vi "GaussianPeakFinder.vi"(3 "Mode":T4, 5 "Traverse line In":T1 {"Row Duration (mins)" format="%#.1f"; "Row No" min=0; "Trace Gas Concentration (%)" min=0.0 format="%#.2f"; "Emission Rate (l/min)" format="%#.2f"; "Tunnel Speed" format="%#.2f"; "Start X" format="%#.2f"; "Start Y" format="%#.2f"; "Start Z" format="%#.2f"; "End X" format="%#.2f"; "End Y" format="%#.2f"; "End Z" format="%#.2f"; "Averaging time (min)" min=0.0 format="%#.2f"}) -> (0 "Error Message":string, 1 "Status":T5, 2 "Traverse line Out":T1 {"Row Duration (mins)" format="%#.1f"; "Row No" min=0; "Trace Gas Concentration (%)" min=0.0 format="%#.2f"; "Emission Rate (l/min)" format="%#.2f"; "Tunnel Speed" format="%#.2f"; "Start X" format="%#.2f"; "Start Y" format="%#.2f"; "Start Z" format="%#.2f"; "End X" format="%#.2f"; "End Y" format="%#.2f"; "End Z" format="%#.2f"; "Averaging time (min)" min=0.0 format="%#.2f"})   [LabVIEW 2011]
uses:
  Gen Trav/Traverse_cluster.ctl
  Gen Trav/Spacing.ctl
  Controls/Multi_run_mode.ctl
  Controls/User_Specific_mode.ctl
  Gen Trav/Multi_Run_Status.ctl
  Controls/Save_Data.ctl
  Controls/Setup.ctl
  Utilities/gaussianFit/GaussianGlobal.vi
panel:
  in  "Tab Control":enum32{"GaussianFitGraph", "RunVINamed"}(tab)
  in  "nPointsInRake":i32=3
  out "nPointsSampled":i32
  in  "SpreadFactor":dbl=0.8
  in  "Turbulence":dbl=0.2
  in  "SampleLengthMultiplier":dbl=2.5
  out "MeasurementCenter":dbl
  # "X           Y            Z"
  # "Start"
  # "End"
  # "X           Y            Z"
  # "Start"
  # "End"
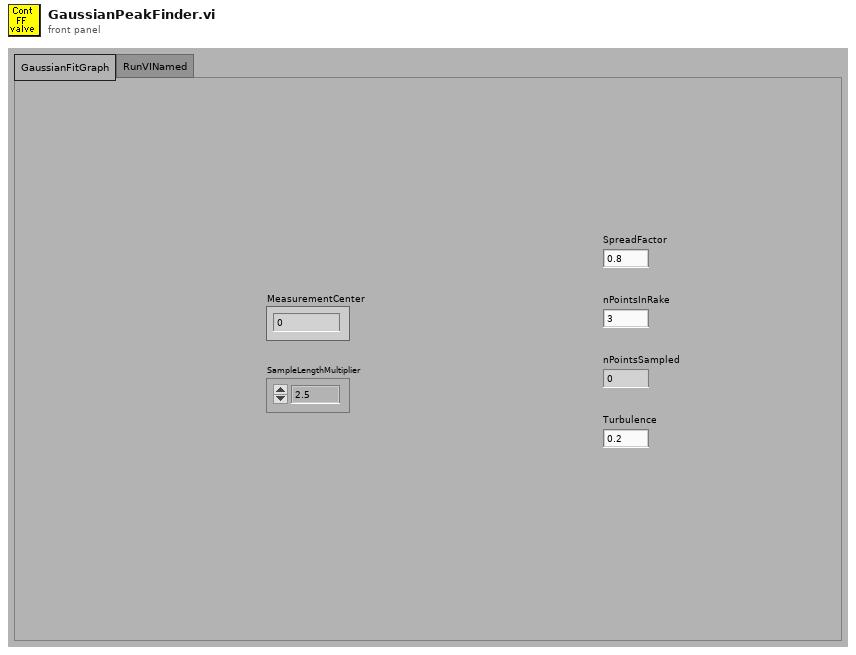
[diagram p1: front panel]
types:
  T1 = typedef "Traverse_cluster.ctl" = cluster{"Start X":dbl, "Start Y":dbl, "Start Z":dbl, "End X":dbl, "End Y":dbl, "End Z":dbl, "No. of pts.":i32, "Spacing":T2, "Filename":path, "Tunnel Speed":dbl, "Averaging time (min)":dbl, "Extra Commands":string, "Specific Arguments":string, "Emission Rate (l/min)":dbl, "Trace Gas Concentration (%)":dbl, "Density Ratio":string, "Comments":string, "Row No":i32, "Row Type Selector":T3, "Completion time":string, "Row Duration (mins)":dbl, "No. of Valid pts.":i32, "Meas Setup File":string}
  T2 = typedef "Spacing.ctl" = enum16{"Linear", "Log", "Gauss", "Specified", "N/A"}
  T3 = typedef "Multi_run_mode.ctl" = enum16{"Move Traverse Only", "Set Tunnel Speed Only", "Set Source Only", "Set Measurement Conditions", "Single Measurement", "Vertical Profile", "Lateral Profile", "Longitudinal Profile", "Explore Volume", "Multi-Axis Profile", "Auto Calibrate", "Meas Fast FID Bkgnd", "Check Beam Power", "Scanning Valve Measurement", "Run VI Named:", "Set ADAM Ch", "Wait (minutes)", "Send Message", "Synchronize With:", "Fall Back to this Row", "Turn Off Row Repeating", "Blank Row", "Traverse 3D Volume"}
  T4 = typedef "User_Specific_mode.ctl" = enum16{"Check VI only", "Run VI"}
  T5 = typedef "Multi_Run_Status.ctl" = enum16{"Continue", "Jump to Next Point", "Jump to Next Row", "Jump To Fall Back", "Terminate Run"}
  T6 = typedef "Save_Data.ctl" = enum16{"Save No Data", "Save Data"}
  T7 = typedef "Setup.ctl" = enum16{"Run Program", "Show Setup", "Save Current Setup", "Setup Front Panel"}
  T8 = typedef "Status_Cluster.ctl" = cluster{"Status":T5, "Error Type":string, "Error Description":string}
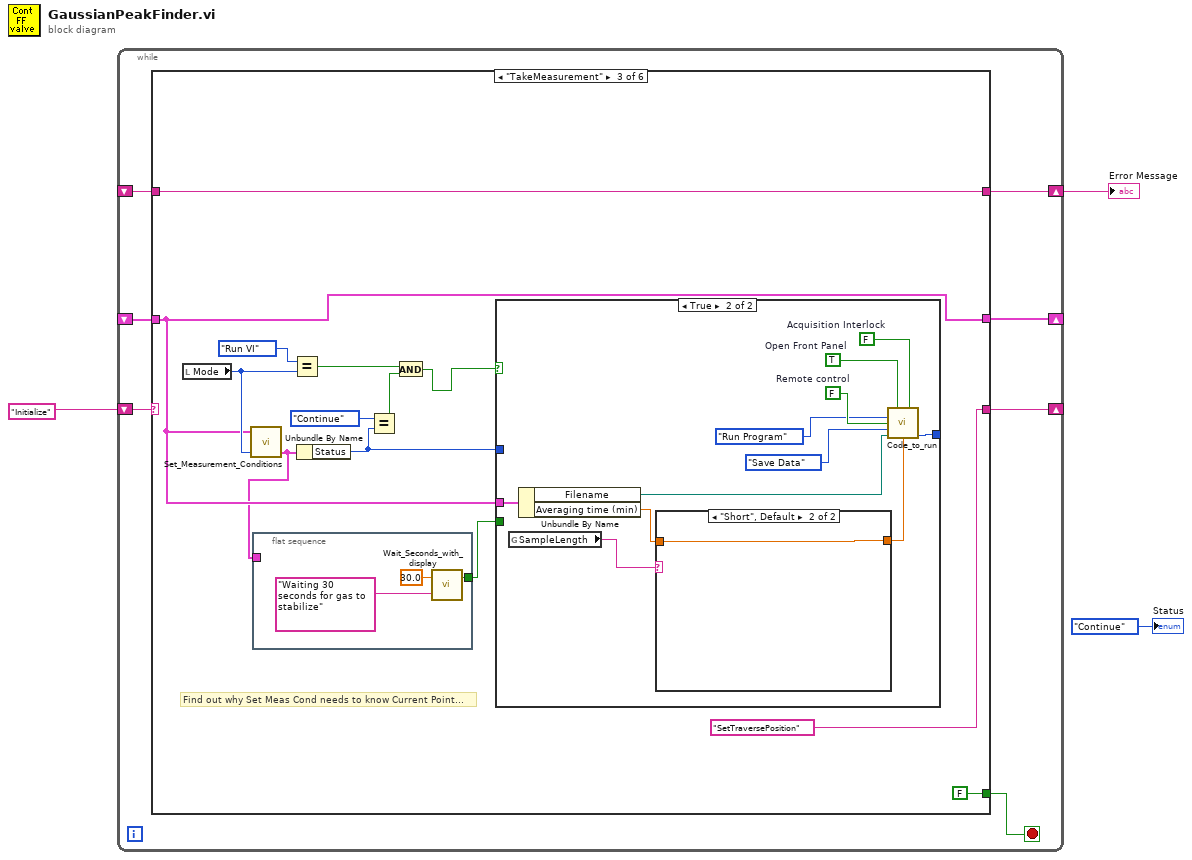
[diagram p0: block diagram]
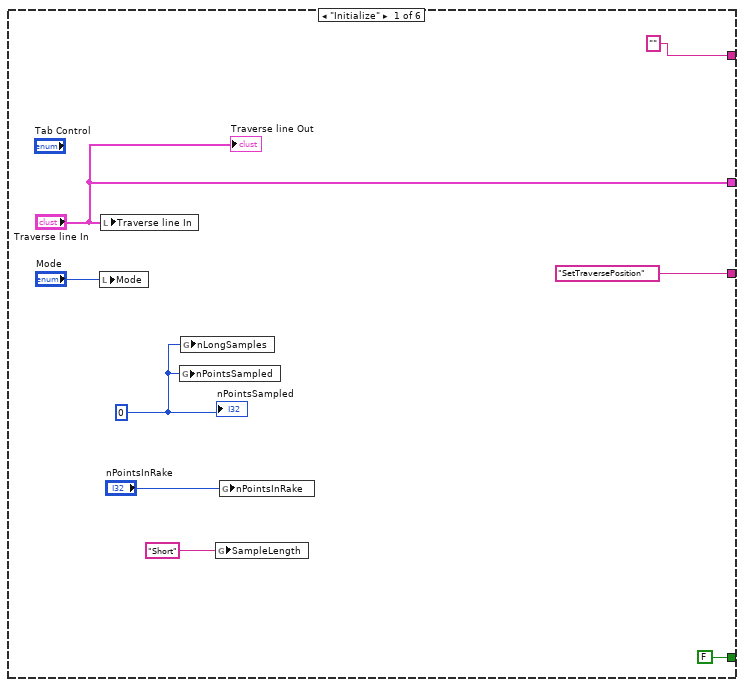
[diagram p2: hidden frame]
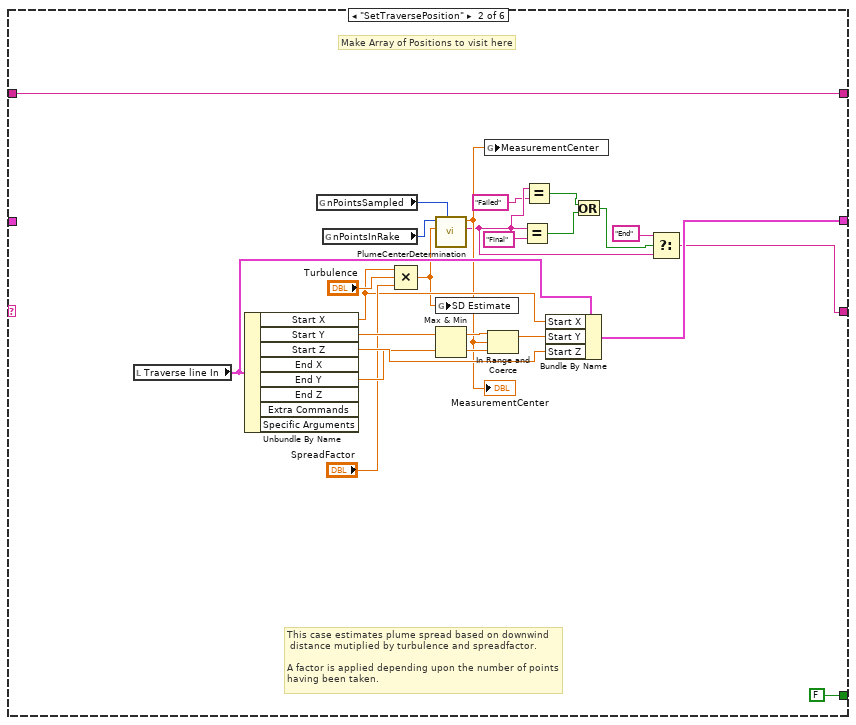
[diagram p3: hidden frame]
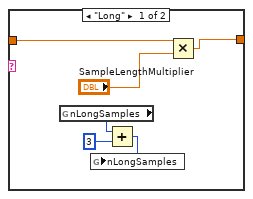
[diagram p5: hidden frame]
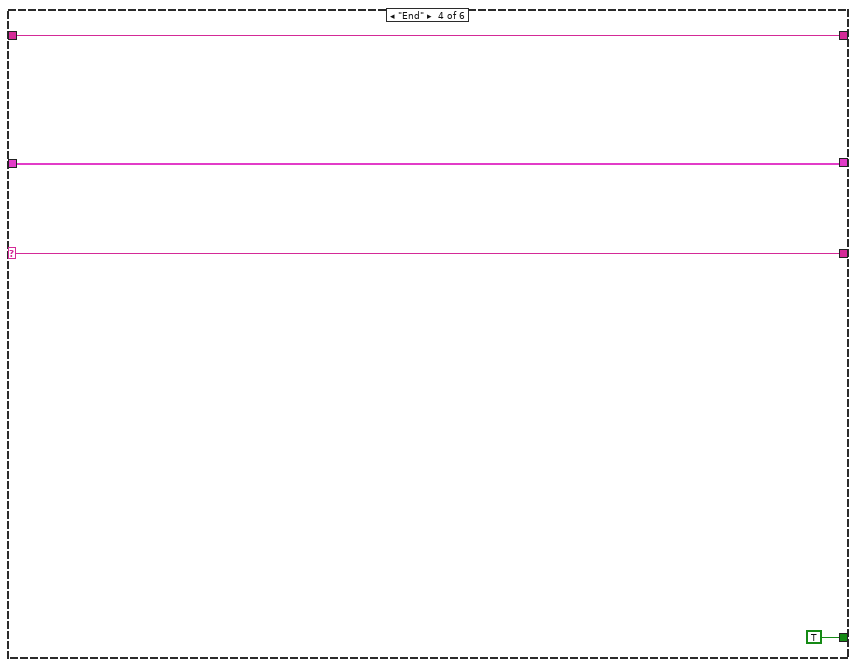
[diagram p6: hidden frame]
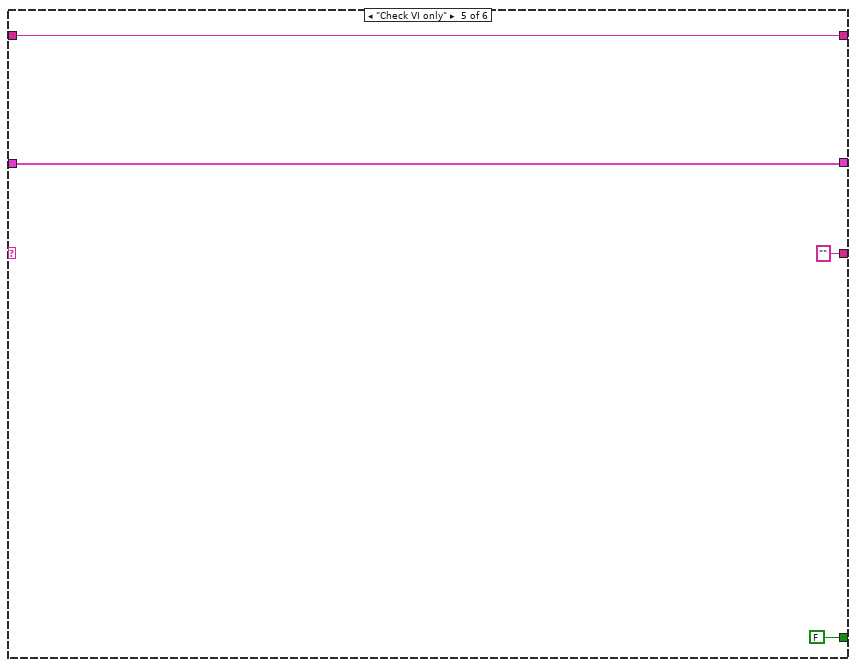
[diagram p7: hidden frame]
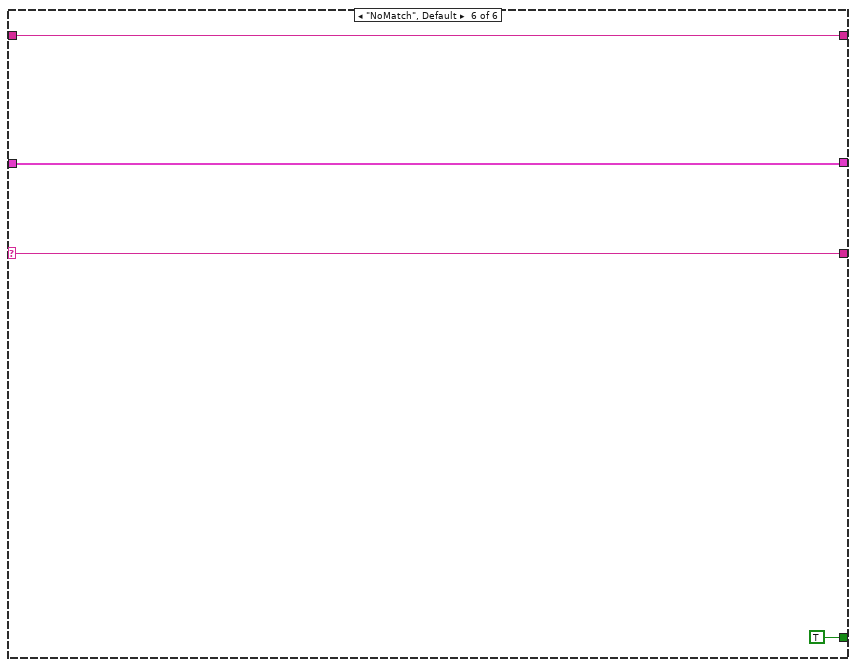
[diagram p8: hidden frame]
diagram:
  n1 = while {
    shift-right: [w8] -> _
    shift-left: _ -> [w7]
    shift-right: [w10] -> w2
    shift-left: _ -> [w5]
    shift-right: [w4] -> _
    shift-left: "Initialize" -> [w9]
    stop <- w6 stop-if-true
    n2 = case shown="\"TakeMeasurement\"" w9 {
      selector: w9 -> [_ _ _ w79 _ w87]
      tunnel: ["" w39 w50 w81 w84 w88] -> w10
      tunnel: ["Traverse line In" w42 w49 w80 w85 w89] -> w8
      tunnel: w7 -> [_ _ w49 w80 w85 w89]
      tunnel: [FALSE FALSE FALSE TRUE FALSE TRUE] -> w6
      tunnel: w5 -> [_ w39 w50 w81 w84 w88]
      tunnel: ["SetTraversePosition" w26 "SetTraversePosition" w79 "" w87] -> w4
      frame "Initialize" {
        w11 = 0 ("PointsSampled")
        n3 = local write "Mode"("Mode") -> ()
        n4 = local write "Traverse line In"("Traverse line In") -> ()
        n5 = global write "GaussianGlobal.vi" "nPointsSampled"(w11) -> ()
        n6 = global write "GaussianGlobal.vi" "nLongSamples"(w11) -> ()
        n7 = global write "GaussianGlobal.vi" "SampleLength"("Short" ("SampleLength")) -> ()
        n8 = global write "GaussianGlobal.vi" "nPointsInRake"("nPointsInRake") -> ()
        "nPointsSampled" <- w11
        "Traverse line Out" <- "Traverse line In"
      }
      frame "SetTraversePosition" {
        # "This case estimates plume spread based on downwind\n distance mutiplied by turbulence and spreadfactor.\n\nA factor is applied depending upon the number of points\nhaving been taken."
        # "Make Array of Positions to visit here"
        n9 = local read "Traverse line In"() -> (w41:T1)
        n10 = Unbundle By Name(w41) -> ("Start X"=w31:dbl, "Start Y"=w38:dbl, "Start Z"=w43:dbl, "End Y"=w37:dbl)  [unwired: 4 out]
        n11 = global read "GaussianGlobal.vi" "nPointsSampled"() -> (w29:i32)
        n12 = global read "GaussianGlobal.vi" "nPointsInRake"() -> (w30:i32)
        n13 = Compound Arithmetic op=MULTIPLY(w31, "Turbulence", "SpreadFactor") -> (w24:dbl)
        n14 = call "PlumeCenterDetermination.vi"("nPointsSampled"=w29, "SD Estimate"=w24, "nPointsInRake"=w30) -> ("CommandString"=w23:string, "Measurement Center"=w25:dbl)  [unwired: 7 in]
        "MeasurementCenter" <- w25
        n15 = global write "GaussianGlobal.vi" "SD Estimate"(w24) -> ()
        n16 = Max & Min(x=w38, y=w37) -> (max(x,y)=w36:dbl, min(x,y)=w35:dbl)
        n17 = global write "GaussianGlobal.vi" "MeasurementCenter"(w25) -> ()
        n18 = In Range and Coerce(upper limit=w36, x=w25, lower limit=w35) -> (coerced(x)=w34:dbl)  [unwired: 1 out]
        n19 = Equal?(x=w23, y="Final") -> (x = y?=w20:bool)
        n20 = Equal?(x=w23, y="Failed") -> (x = y?=w21:bool)
        n21 = Bundle By Name(cluster=w41, "Start X"=w31, "Start Y"=w34, "Start Z"=w43) -> (w42:T1)
        n22 = Or(x=w21, y=w20) -> (x .or. y?=w19:bool)
        n23 = Select(t="End" ("y"), s=w19, f=w23) -> (s? t:f=w26:string)
      }
      frame "TakeMeasurement" {
        # "Find out why Set Meas Cond needs to know Current Point..."
        n24 = local read "Mode"() -> (w52:T4)
        n25 = call "Set_Measurement_Conditions.vi"("Simulate/Run"=w52, "Traverse line"=w49) -> ("Status Cluster"=w44:T8)  [unwired: 3 in]
        n26 = flat-sequence {
          tunnel: [w59] -> w46
          tunnel: w44 -> [_]
          frame #0 {
            n27 = call "Wait_Seconds_with_display.vi"("Message"="Waiting 30 seconds for gas to stabilize", "Seconds to wait"=30.0) -> ("Stopped"=w59:bool)  [unwired: 1 in]
          }
        }
        n28 = Equal?(x=User_Specific_mode."Run VI" ("Mode"), y=w52) -> (x = y?=w56:bool)
        n29 = Unbundle By Name(w44) -> ("Status"=w47:T5)
        n30 = Equal?(x=Multi_Run_Status."Continue" ("Status"), y=w47) -> (x = y?=w53:bool)
        n31 = And(x=w56, y=w53) -> (x .and. y?=w45:bool)
        n32 = case shown="True" w45 {
          tunnel: w49 -> [_ w71]
          tunnel: w47 -> [w60 _]
          tunnel: [w60 w65] -> _
          tunnel: w46 -> [_ _]
          frame False {
          }
          frame True {
            w68 = FALSE  # Acquisition Interlock
            w69 = TRUE  # Open Front Panel
            w70 = FALSE  # Remote control
            n33 = global read "GaussianGlobal.vi" "SampleLength"() -> (w63:string)
            n34 = Unbundle By Name(w71) -> ("Filename"=w64:path, "Averaging time (min)"=w62:dbl)
            n35 = case shown="\"Short\", Default" w63 {
              tunnel: w62 -> [w77 w78]
              tunnel: [w75 w78] -> w61
              frame "Long" {
                n36 = global read "GaussianGlobal.vi" "nLongSamples"() -> (w72:i32)
                n37 = Add(x=w72, y=3) -> (x+y=w73:i32)
                n38 = global write "GaussianGlobal.vi" "nLongSamples"(w73) -> ()
                n39 = Multiply(x=w77, y="SampleLengthMultiplier") -> (x*y=w75:dbl)
              }
              frame "Short", Default {
              }
            }
            n40 = call "Code_to_run.vi"("Open Front Panel"=w69, "Acquisition Interlock"=w68, "setup"=Setup."Run Program", "Remote control"=w70, "File"=Save_Data."Save Data", "Results Filename"=w64, "Averaging time (min)"=w61) -> ("Status"=w65:T5)  [unwired: 8 in]
          }
        }
      }
      frame "End" {
      }
      frame "Check VI only" {
      }
      frame "NoMatch", Default {
      }
    }
  }
  "Error Message" <- w2
  "Status" <- Multi_Run_Status."Continue" ("Status")
